vi "GoHome.vi"(4 "Home fail":refnum<vi>, 6 "HomeDone":refnum<vi>, 7 "Busy":refnum<vi>, 8 "error in (no error)":errorcluster, 11 "Motor in":refnum<class "Motor.lvclass">) -> (0 "error out":errorcluster, 2 "String":string, 3 "Motor out":refnum<class "Motor.lvclass">)   [LabVIEW 2018, in "Motor.lvclass"]
uses:
  Motor.lvclass
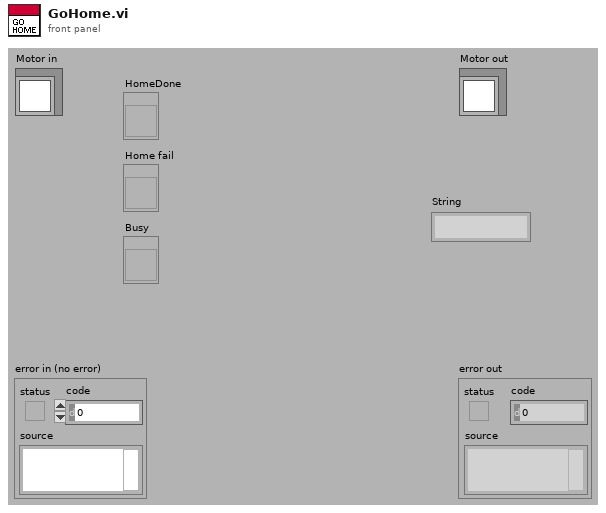
[diagram p1: front panel]
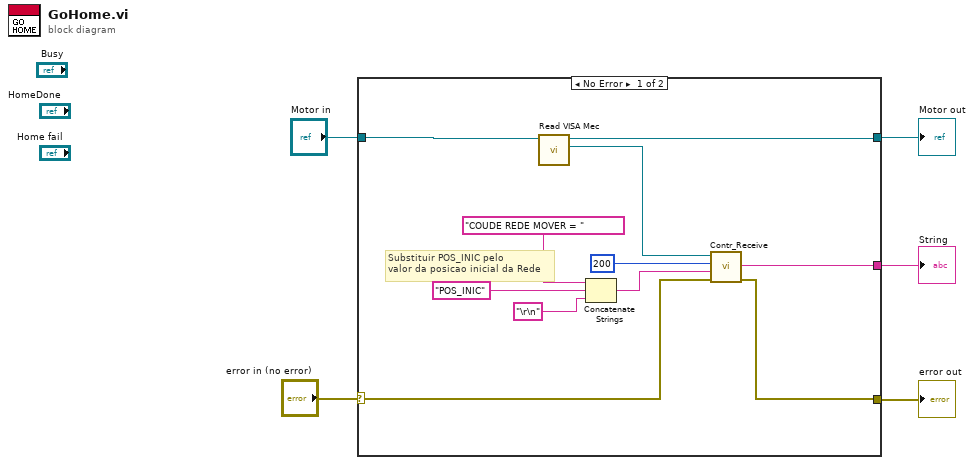
[diagram p0: block diagram]
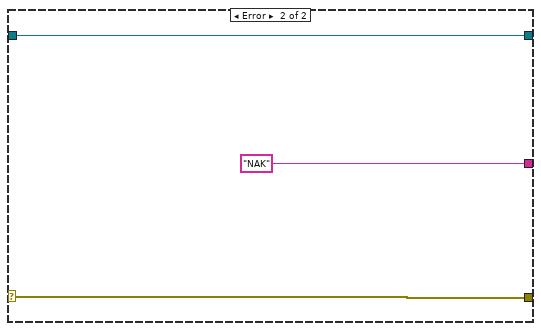
[diagram p2: hidden frame]
diagram:
  n1 = case shown="No Error" "error in (no error)" {
    selector: "error in (no error)" -> [w11 w17]
    tunnel: "Motor in" -> [w10 w18]
    tunnel: [w9 w18] -> w3
    tunnel: [w8 w17] -> w2
    tunnel: [w7 "NAK"] -> w1
    frame No Error {
      # "Substituir POS_INIC pelo\nvalor da posicao inicial da Rede"
      n2 = call-dynamic "Read VISA Mec.vi"("Controlador in"=w10) -> ("VISA Mec"=w15:refnum<visa-resource-name>, "Controlador out"=w9:refnum<class "Motor.lvclass">)  [unwired: 8 in, 1 out]
      n3 = Concatenate Strings("COUDE REDE MOVER = " ("Command to SIFS"), "POS_INIC" ("string"), "\r\n" ("string")) -> (w12:string)
      n4 = call "Contr_Receive.vi"("error in"=w11, "Command to SIFS"=w12, "wait after tx"=u32 200, "VISA resource name"=w15) -> ("error out"=w8:errorcluster, "Response from SIFS"=w7:string)  [unwired: 2 out]
    }
    frame Error {
    }
  }
  "error out" <- w2
  "Motor out" <- w3
  "String" <- w1
